vi "rx_projvi.vi"() -> ()   [LabVIEW 2023]
uses:
  <vilib>/addons/Modulation/Analog/support/mod_Set Error Source.vi
  <vilib>/addons/Modulation/Digital/Support/Common/Validators/mod_Generate Filter Coefficients Validate.vi
  <vilib>/addons/Modulation/Digital/General/subVIs/mod_Generate Filter Coefficients.vi
  <vilib>/addons/Modulation/Digital/General/MT Generate QAM System Parameters(M).vi
  <instrlib>/niUSRP/niUSRP Fetch Rx Data (CDB Cluster).vi
  <vilib>/addons/Modulation/niDMT.lvlib
panel:
  out "constellation graph 4":T1(array[cluster]) {"oversampled data" format="%.2f"; "constellation" format="%.2f"}
  out "Rx Const 2":T1(graph)
  in  "samples per symbol (16) 2":i32=16
  in  "filter parameter 2":dbl=0.5 format="%.2f"
  in  "matched samples per symbol (16) 2":i32=16
  in  "pulse shaping samples per symbol (16) 2":i32=16
  in  "M-QAM (16) 2":i32=16
  in  "pulse shaping filter (none) 2":T2(ring)
  out "Demodulated 2":cluster{"t0":dbl, "dt":dbl, "Y":dbl[]}(graph)
  out "coerced gain":dbl format="%#_6f"
  out "coerced carrier frequency":dbl=100000.0 format="%#_6p"
  out "coerced IQ rate":dbl=100000.0 format="%#_6p"
  in  "Recv carrier frequency":dbl=100000.0 format="%#_6p"
  in  "Recv IQ rate":dbl=100000.0 format="%#_6p"
  in  "number of samples":i64=100000
  in  "stop 2":bool
  in  "active antenna 2":string
  in  "gain":dbl format="%#_6f"
  out "error out 2":errorcluster
  in  "error in (no error)":errorcluster
  in  "USRP IP Address":refnum<k15>
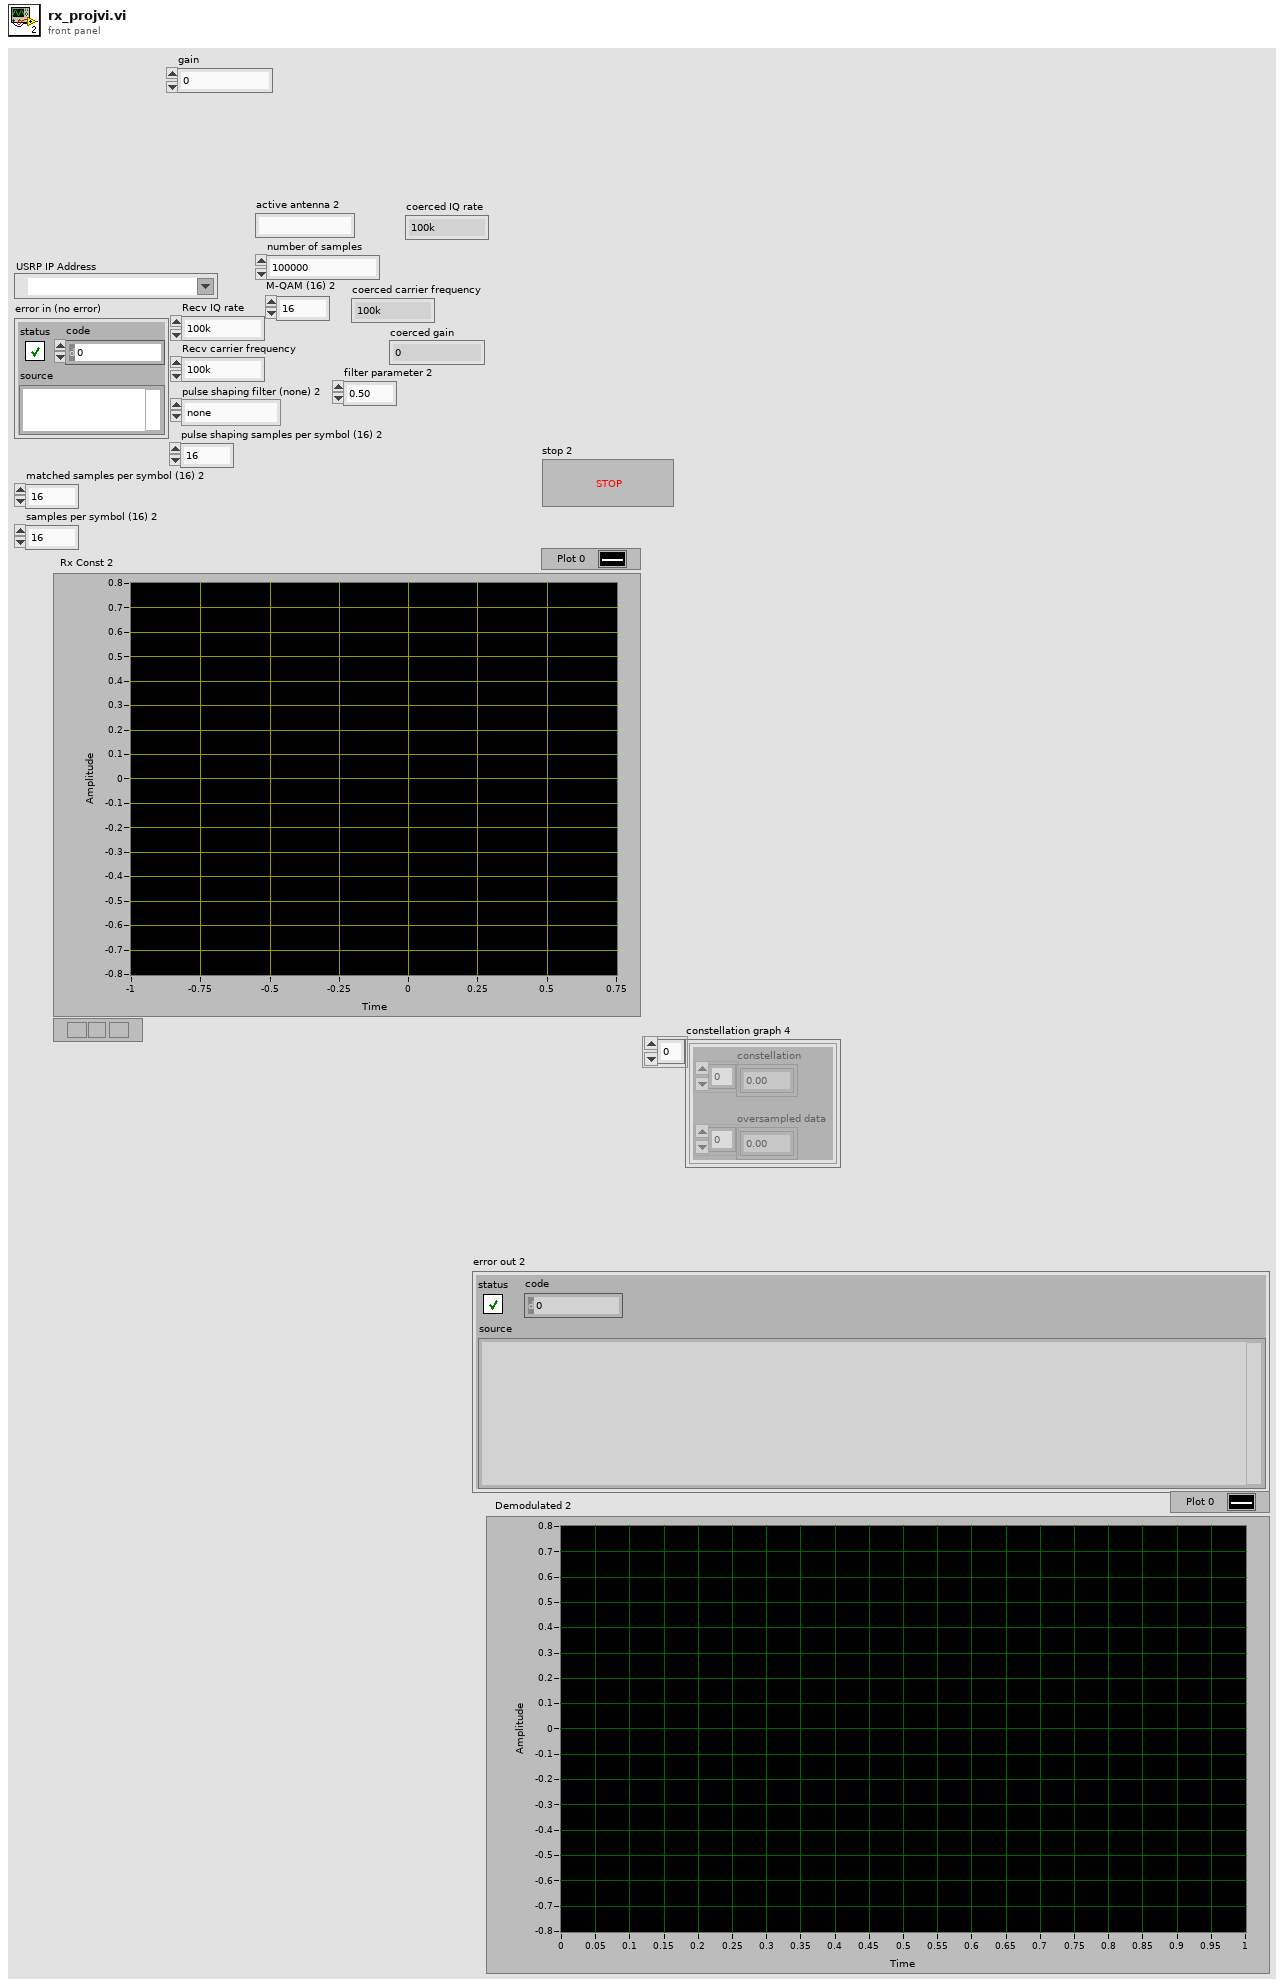
[diagram p1: front panel]
types:
  T1 = cluster{"constellation":dbl[], "oversampled data":dbl[]}[]
  T2 = enum16{"none", "Raised Cosine", "Root Raised Cos", "Gaussian"}
  T3 = enum16{"FSK", "PSK", "QAM", "MSK", "PAM", "ASK", "CPM"}
  T4 = cluster{"samples per symbol (16)":i32, "symbol map":cdb[]}
  T5 = typedef "niAMT.lvlib/Complex Data Waveform.ctl" = cluster{"t0":dbl, "dt":dbl, "Y":cdb[]}
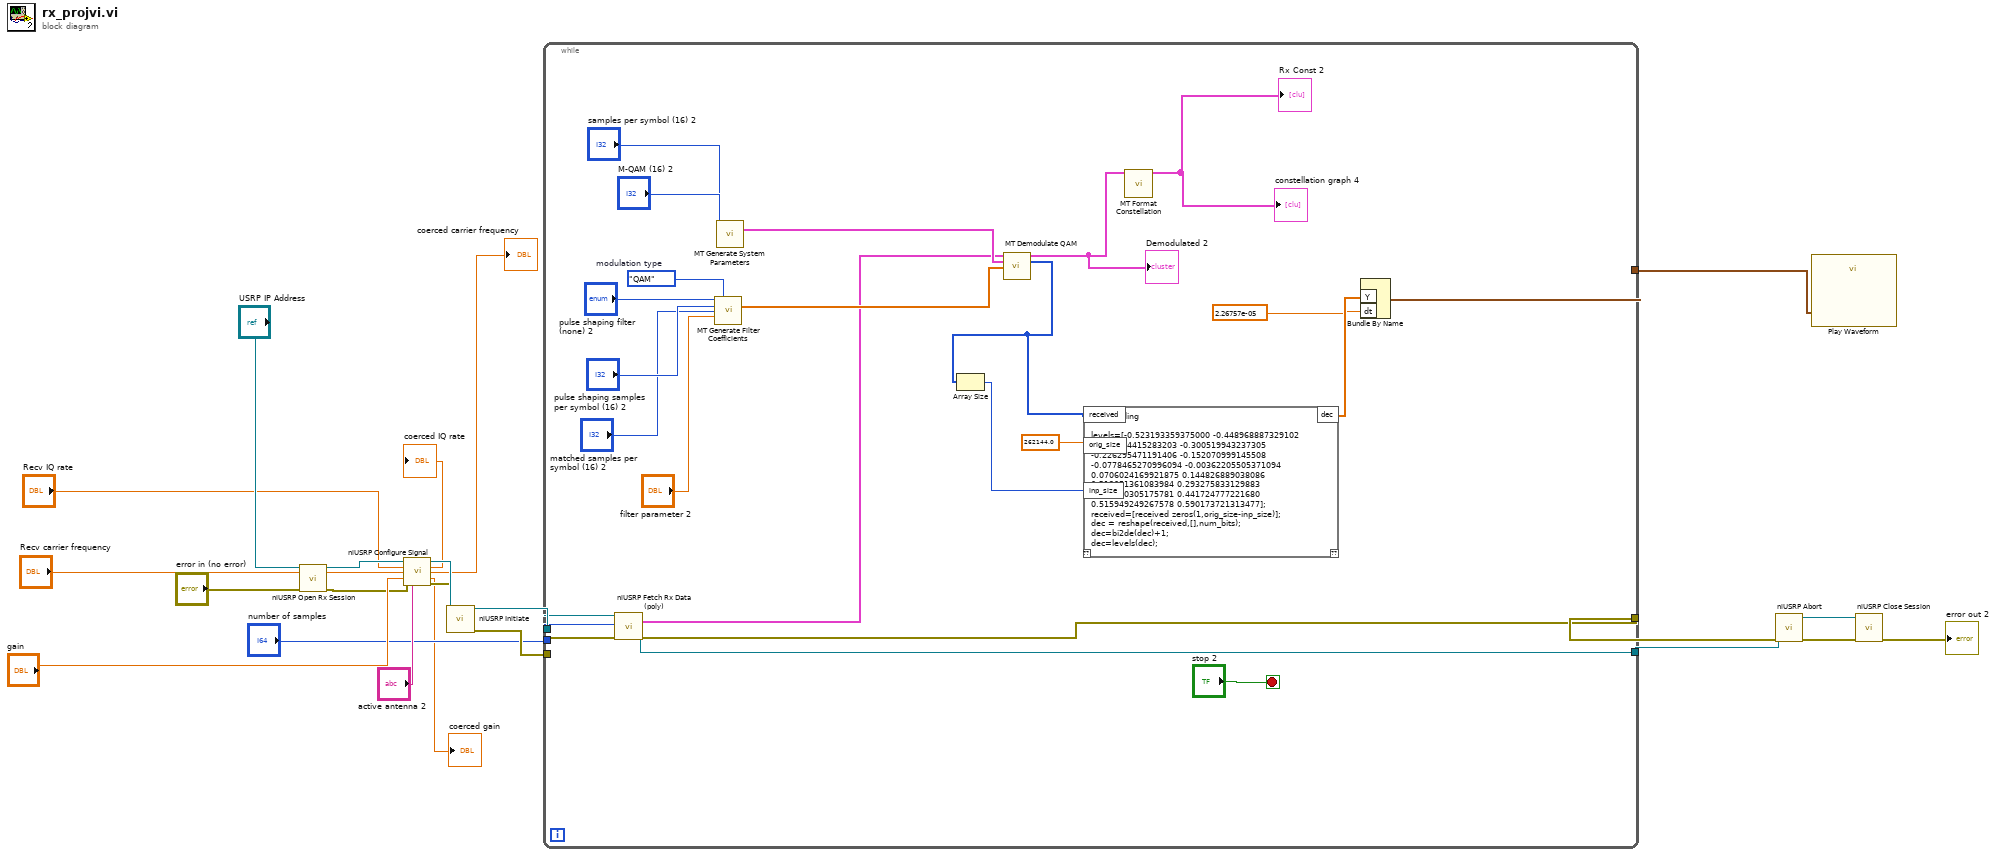
[diagram p0: block diagram]
diagram:
  n1 = call <instrlib>:"niUSRP Open Rx Session.vi"("device names"="USRP IP Address", "error in (no error)"="error in (no error)") -> ("session handle out"=w20:refnum<k15>, "error out"=w2:errorcluster)  [unwired: 12 in]
  n2 = call <instrlib>:"niUSRP Configure Signal.vi"("session handle"=w20, "IQ rate"="Recv IQ rate", "carrier frequency"="Recv carrier frequency", "gain"="gain", "error in (no error)"=w2, "active antenna"="active antenna 2") -> ("session handle out"=w17:refnum<k15>, "coerced IQ rate"=→"coerced IQ rate":dbl, "coerced carrier frequency"=→"coerced carrier frequency":dbl, "coerced gain"=→"coerced gain":dbl, "error out"=w16:errorcluster)  [unwired: 5 in]
  n3 = call <instrlib>:"niUSRP Initiate.vi"("session handle"=w17, "error in (no error)"=w16) -> ("session handle out"=w15:refnum<k15>, "error out"=w14:errorcluster)  [unwired: 12 in]
  n4 = while {
    tunnel: w15 -> [w46]
    tunnel: w14 -> [w45]
    tunnel: "number of samples" -> [w41]
    tunnel: [w44] -> w5
    tunnel: [w43] -> w4
    tunnel: [w23] -> w1
    stop <- "stop 2" stop-if-true
    w40 = T3."QAM"  # modulation type
    n5 = call-poly <instrlib>:"niUSRP Fetch Rx Data (poly).vi"("session handle"=w46, "number of samples"=w41, "error in (no error)"=w45) -> ("session handle out"=w44:refnum<k15>, "data"=w25:cluster{"t0":dbl, "dt":dbl, "Y":cdb[]}, "error out"=w43:errorcluster)  [unwired: 9 in, 1 out]
    n6 = call <vilib>:"MT Generate Filter Coefficients.vi"("pulse shaping filter (none)"="pulse shaping filter (none) 2", "modulation type"=w40, "pulse shaping samples per symbol (16)"="pulse shaping samples per symbol (16) 2", "matched samples per symbol (16)"="matched samples per symbol (16) 2", "filter parameter"="filter parameter 2") -> ("matched filter coefficients"=w32:dbl[])  [unwired: 8 in, 2 out]
    n7 = call-poly <vilib>:"MT Generate System Parameters.vi"("samples per symbol (16)"="samples per symbol (16) 2", "M-QAM (16)"="M-QAM (16) 2") -> ("QAM system parameters"=w33:T4)  [unwired: 11 in, 2 out]
    n8 = call <vilib>:"MT Demodulate QAM.vi"("input complex waveform"=w25, "QAM system parameters"=w33, "matched filter coefficients"=w32) -> ("recovered complex waveform"=w30:T5, "output bit stream"=w29:i8[])  [unwired: 8 in, 3 out]
    "Demodulated 2" <- w30
    n9 = Array Size(array=w29) -> (size(s)=w27:i32)
    n10 = script code="% Decoding \n\nlevels=[-0.523193359375000\t-0.448968887329102\t-0.374744415283203\t-0.300519943237305\t-0.226295471191406\t-0.152070999145508\t-0.0778465270996094\t-0.00362205505371094\t0.0706024169921875\t0.144826889038086\t0.219051361083984\t0.293275833129883\t0.367500305175781\t0.441724777221680\t0.515949249267578\t0.590173721313477];\nreceived=[received zeros(1,orig_size-inp_size)];\ndec = reshape(received,[],num_bits);\ndec=bi2de(dec)+1;\ndec=levels(dec);"("received"=w29, "inp_size"=w27, "orig_size"=262144.0 ("Real")) -> ("dec"=w26:dbl[])  [unwired: 1 in, 1 out]
    n11 = call <vilib>:"MT Format Constellation.vi"("waveform"=w30) -> ("constellation graph"=→"Rx Const 2" →"constellation graph 4":T1)  [unwired: 13 in, 1 out]
    n12 = Bundle By Name("Y"=w26, "dt"=2.26757e-05) -> (w23:waveform(dbl))  [unwired: 1 in]
  }
  n13 = call <instrlib>:"niUSRP Abort.vi"("session handle"=w5, "error in (no error)"=w4) -> ("session handle out"=w12:refnum<k15>, "error out"=w11:errorcluster)  [unwired: 12 in]
  n14 = call "Play Waveform"("Data"=w1) -> ()  [unwired: 18 in, 1 out]
  n15 = call <instrlib>:"niUSRP Close Session.vi"("session handle"=w12, "error in (no error)"=w11) -> ("error out"=→"error out 2":errorcluster)  [unwired: 13 in]
